vi "UpdateBlockData.vi"(5 "BlockUpdate":bool, 6 "singleDirectionScan":bool, 7 "Data":sgl[](array[numeric]), 8 "Lines":u32, 9 "linesPerUpdate":u16, 10 "ScanEnable?":bool, 11 "Pixels/Line":u32) -> (0 "current time":timestamp, 1 "LineIndex":u32, 4 "EndOfScan?":bool)   [LabVIEW 2016]
uses:
  controls/Enum.ctl
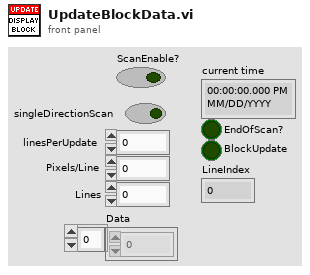
[diagram p1: front panel]
types:
  T1 = typedef "Enum.ctl" = enum16{"Init", "Read", "Write"}
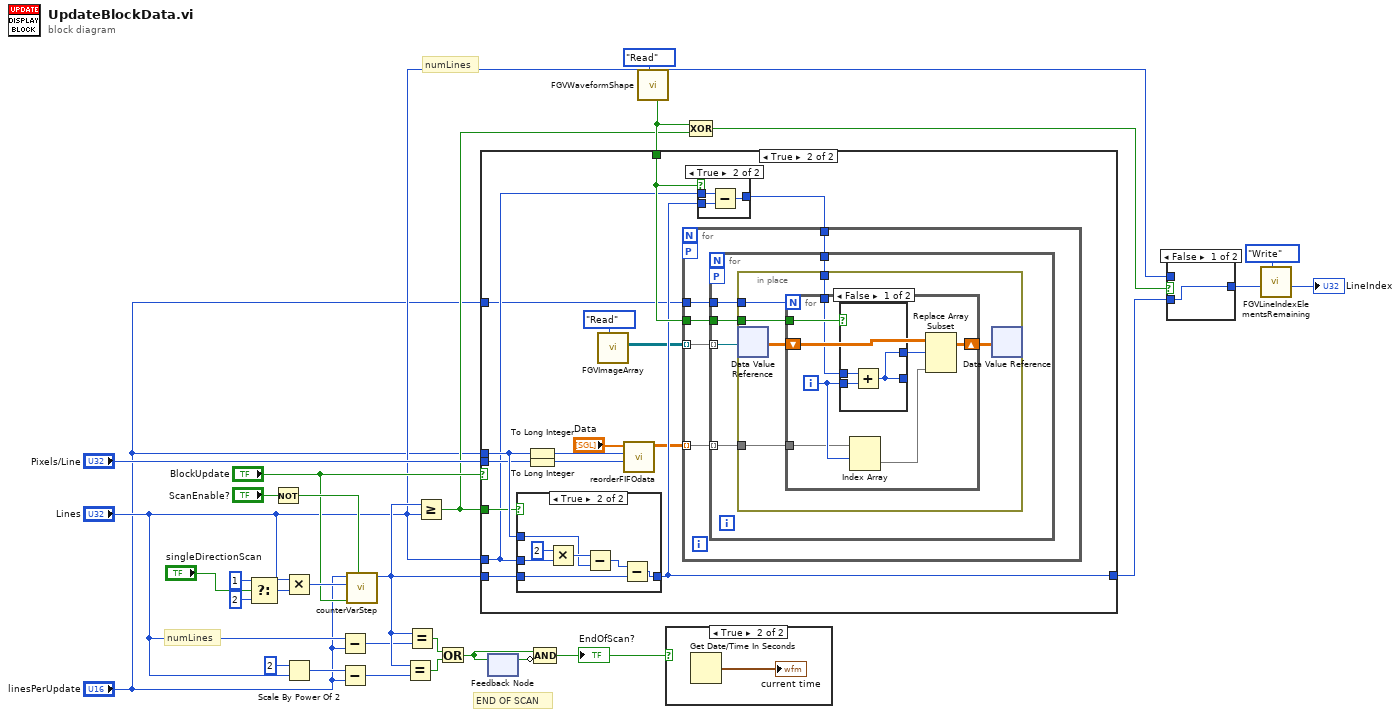
[diagram p0: block diagram]
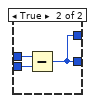
[diagram p3: hidden frame]
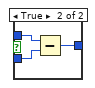
[diagram p6: hidden frame]
diagram:
  # "numLines"
  # "numLines"
  # "END OF SCAN"
  n1 = Select(t=u16 1, s="singleDirectionScan", f=u16 2 ("y")) -> (s? t:f=w27:u16)
  n2 = Not(x="ScanEnable?") -> (.not. x?=w29:bool)
  n3 = Multiply(x="Lines", y=w27) -> (x*y=w18:u32)
  n4 = Scale By Power Of 2(n=i16 2, x="Lines") -> (x*2^n=w23:u32)
  n5 = Subtract(x="Lines", y="linesPerUpdate") -> (x-y=w21:u32)
  n6 = Subtract(x=w23, y="linesPerUpdate") -> (x-y=w24:u32)
  n7 = call "counterVarStep.vi"("stepSize"="linesPerUpdate", "countMax"=w18, "doStep"="BlockUpdate", "reset"=w29) -> ("index"=w28:u32)  [unwired: 4 in, 2 out]
  n8 = Equal?(x=w28, y=w24) -> (x = y?=w20:bool)
  n9 = Equal?(x=w28, y=w21) -> (x = y?=w19:bool)
  n10 = Greater Or Equal?(x=w28, y="Lines") -> (x >= y?=w9:bool)
  n11 = Or(x=w19, y=w20) -> (x .or. y?=w5:bool)
  n12 = feedback #1() -> (w25:bool)  [unwired: 1 in]
  n13 = feedback-in #1(w5) -> ()
  n14 = Compound Arithmetic op=AND(w5, invert w25) -> (w13:bool)
  "EndOfScan?" <- w13
  n15 = call "FGVWaveformShape.vi"("Enum"=Enum."Read") -> ("Framing up? (down: f) out"=w10:bool)  [unwired: 6 in, 4 out]
  n16 = case shown="True" "BlockUpdate" {
    tunnel: "linesPerUpdate" -> [_ w45]
    tunnel: "Pixels/Line" -> [_ w44]
    tunnel: w28 -> [w30 w43]
    tunnel: "Lines" -> [_ w40]
    tunnel: [w30 w39] -> w11
    tunnel: w10 -> [_ w41]
    tunnel: w9 -> [_ w42]
    tunnel: "linesPerUpdate" -> [_ w32]
    frame False {
    }
    frame True {
      n17 = case shown="True" w42 {
        tunnel: [w80 w85] -> w39
        tunnel: w45 -> [_ w83]
        tunnel: w43 -> [w80 w82]
        tunnel: w40 -> [_ w81]
        frame False {
        }
        frame True {
          n18 = Multiply(x=u32 2, y=w81) -> (x*y=w86:u32)
          n19 = Subtract(x=w86, y=w83) -> (x-y=w84:u32)
          n20 = Subtract(x=w84, y=w82) -> (x-y=w85:u32)
        }
      }
      n21 = To Long Integer(number=w45) -> (32bit integer=w38:i32)
      n22 = To Long Integer(number=w44) -> (32bit integer=w37:i32)
      n23 = call "FGVImageArray.vi"("Enum"=Enum."Read") -> ("ImageRefOut"=w33:refnum<data-value>[][])  [unwired: 9 in, 1 out]
      n24 = call "reorderFIFOdata.vi"("pointsPerLine"=w37, "numLines"=w38, "inputElements"="Data") -> ("Reshaped"=w31:sgl[][][][])  [unwired: 8 in]
      n25 = case shown="True" w41 {
        tunnel: w40 -> [_ w79]
        tunnel: w39 -> [w76 w78]
        tunnel: [w76 w77] -> w36
        frame False {
        }
        frame True {
          n26 = Subtract(x=w79, y=w78) -> (x-y=w77:u32)
        }
      }
      n27 = for {
        tunnel: w33 -> [w50] mode=indexing
        tunnel: w41 -> [w49]
        tunnel: w36 -> [w48]
        tunnel: w32 -> [w47]
        tunnel: w31 -> [w46] mode=indexing
        workers-P: _ -> [_]
        n28 = for {
          tunnel: w50 -> [w54] mode=indexing
          tunnel: w49 -> [w55]
          tunnel: w48 -> [w53]
          tunnel: w47 -> [w52]
          tunnel: w46 -> [w51] mode=indexing
          workers-P: _ -> [_]
          n29 = in-place {
            in-place-border: w55 -> [w59]
            in-place-border: w53 -> [w61]
            in-place-border: w52 -> [w58]
            in-place-border: w51 -> [w57]
            n30 = in-place-dvr #2(w54) -> (w60:sgl[][])  [unwired: 1 out]
            n31 = for {
              N: w58 -> [_]
              tunnel: w61 -> [w64]
              tunnel: w59 -> [w69]
              shift-right: [w67] -> w56
              shift-left: w60 -> [w68]
              tunnel: w57 -> [w62]
              i -> [w65]
              n32 = case shown="False" w69 {
                tunnel: w64 -> [w72 w74]
                tunnel: w65 -> [w71 w75]
                tunnel: [w70 w73] -> w63
                tunnel: [w70 w73] -> _
                frame False {
                  n33 = Add(x=w72, y=w71) -> (x+y=w70:u32)
                }
                frame True {
                  n34 = Subtract(x=w74, y=w75) -> (x-y=w73:u32)
                }
              }
              n35 = Index Array(array=w62, index (row)=w65) -> (element=w66:sgl[])  [unwired: 1 in]
              n36 = Replace Array Subset(array=w68, new element=w66, index (row)=w63) -> (w67:sgl[][])  [unwired: 1 in]
            }
            n37 = in-place-dvr #2(w56) -> ()  [unwired: 2 out]
          }
        }
      }
    }
  }
  n38 = case shown="True" w13 {
    frame False {
    }
    frame True {
      n39 = Get Date/Time In Seconds() -> (seconds since 1Jan1904=→"current time":timestamp)
    }
  }
  n40 = Compound Arithmetic op=XOR(w10, w9) -> (w8:bool)
  n41 = case shown="False" w8 {
    tunnel: "Lines" -> [_ w91]
    tunnel: w11 -> [w89 w90]
    tunnel: [w89 w92] -> w2
    frame False {
    }
    frame True {
      n42 = Subtract(x=w91, y=w90) -> (x-y=w92:u32)
    }
  }
  n43 = call "FGVLineIndexElementsRemaining.vi"("Enum"=Enum."Write", "lineIndexIn"=w2) -> ("lineIndexOut"=→"LineIndex":u32)  [unwired: 8 in, 1 out]
